vi "Qrcode Enum Page.vi"() -> ()   [LabVIEW 2019]
uses:
  <vilib>/userDefined/High Color/IMAQdx.ctl
  <vilib>/vision/driver/NI_Vision_Acquisition_Software.lvlib
  <vilib>/vision/NI_Vision_Development_Module.lvlib
panel:
  out "Page 2":string[](array[string])
  out "Page 1":string[](array[string])
  out "SIze Page 2":i32
  out "Size Page 1":i32
  out "Output Enum Data":enum16{"Page 1", "Page 2"}(ring)
  out "Index":i32
  in  "Enum Data":enum16{"Page 1", "Page 2"}[](array[ring])
  out "Data":string
  out "Array":string[](array[string])
  in  "Tab Control":enum32{"Data Qrcode", "Page 1", "Page 2"}(tab)
  out "Data Qrcode":string[](array[string])
  out "Found?":bool
  in  "Session In":T1
  out "Image":T2(plugin-control)
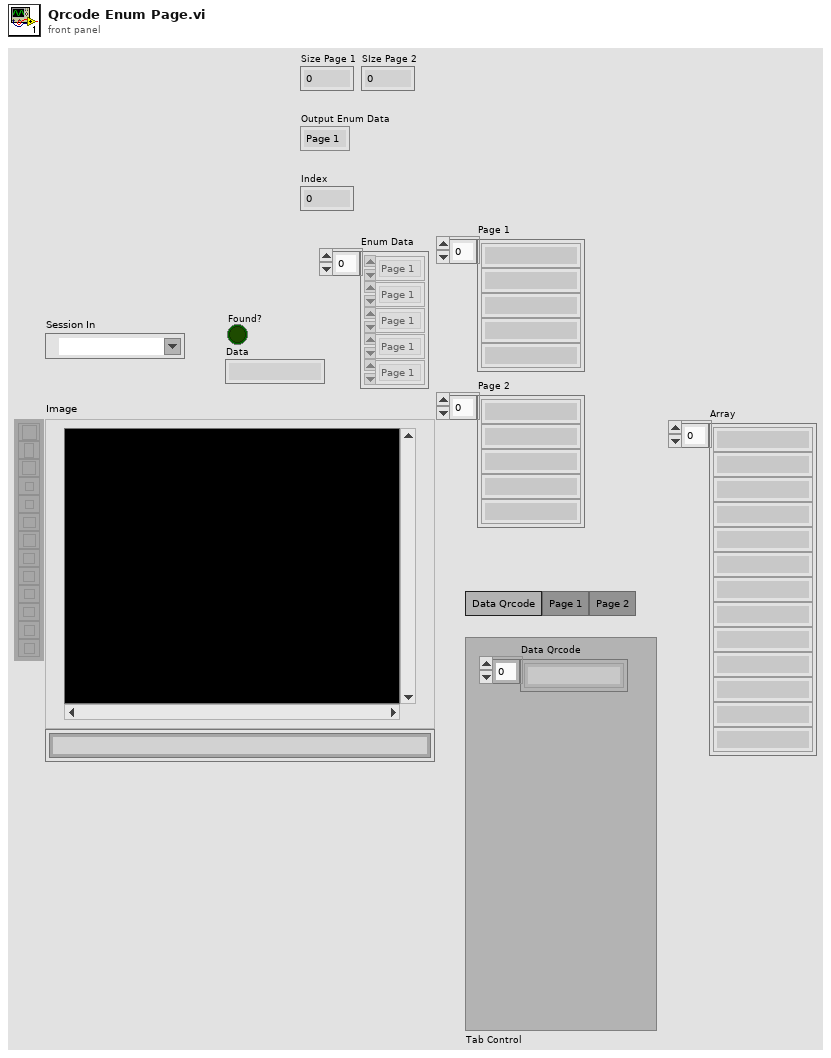
[diagram p1: front panel]
types:
  T1 = typedef "IMAQdx.ctl" = refnum<k21>
  T2 = typedef "IMAQ Image.ctl" = refnum<image>
  T3 = typedef "Image Type" = u32
  T4 = typedef "QR Code Report.ctl" = cluster{"Found?":bool, "Data":string, "Bounding Box":cluster{"x":sgl, "y":sgl}[], "Errors Corrected":u32, "Dimensions (Rows/Cols)":u32, "Version":u32, "QR Model":T5, "Stream Mode":T6, "Barcode Polarity":T7, "Mirrored?":bool, "Append Stream Position":u32, "Size of Append Stream":u32, "First EAN-128 ID":i32, "First Alternate Language ID":i32, "Append Stream ID":u32, "Minimum Edge Strength":u32, "Demodulation Mode":T8, "Cell Sample Size":T9, "Cell Filter Mode":T10}
  T5 = typedef "QR Code Model Type.ctl" = i32
  T6 = typedef "QR Code Stream Mode Type.ctl" = i32
  T7 = typedef "Data Matrix Polarity.ctl" = i32
  T8 = typedef "Demodulation Mode.ctl" = i32
  T9 = typedef "Cell Sample Size.ctl" = i32
  T10 = typedef "Cell Filter Mode.ctl" = i32
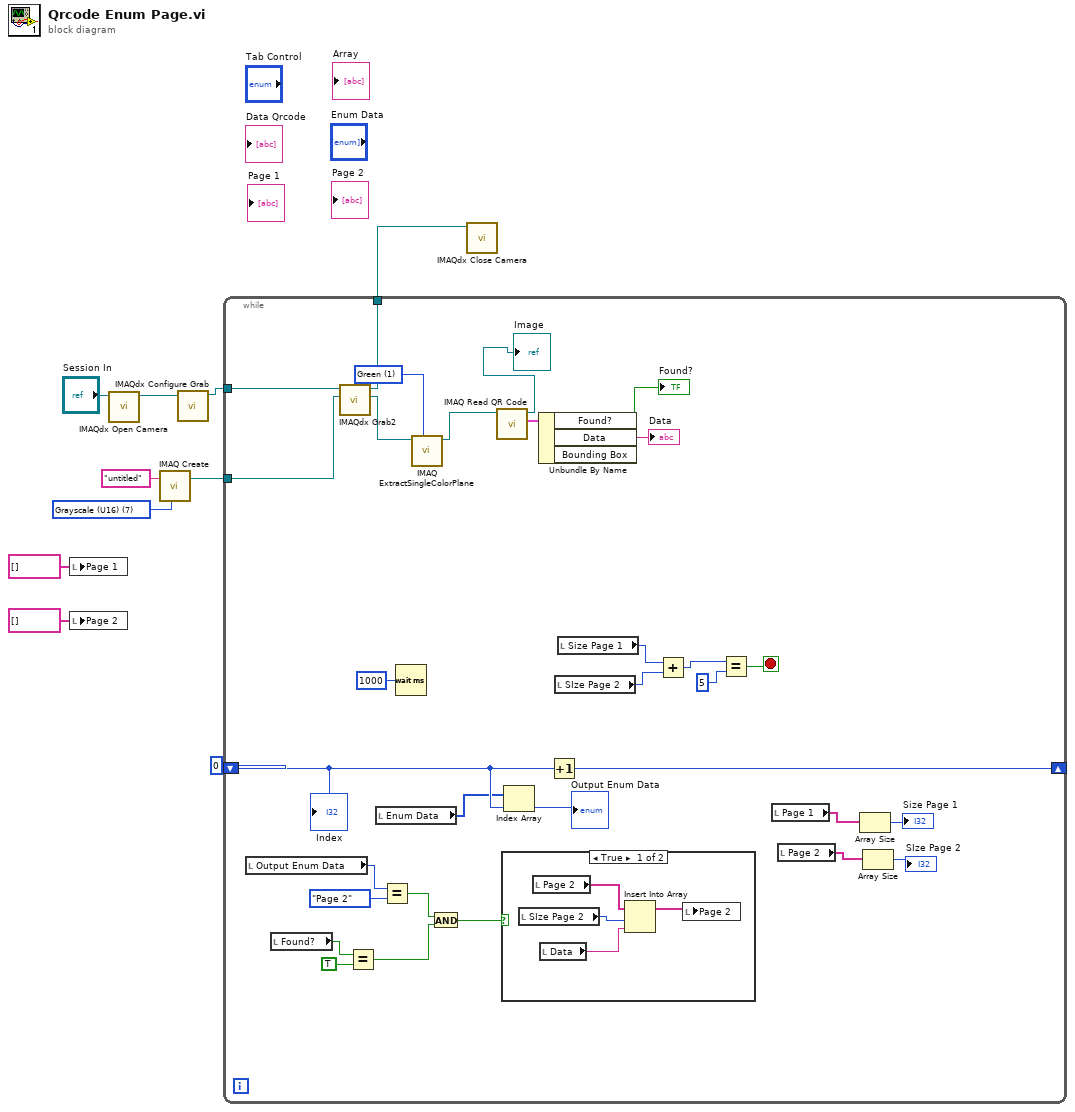
[diagram p0: block diagram]
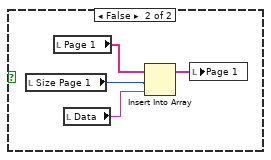
[diagram p2: hidden frame]
diagram:
  w9 = T3 7 items=["Grayscale (U8)", "Grayscale (I16)", "Grayscale (SGL)", "Complex (CSG)", "RGB (U32)", "HSL (U32)", "RGB (U64)", "Grayscale (U16)"] ("Image Type")
  n1 = local write "Page 1"(string[] [] ("Page 1")) -> ()
  n2 = local write "Page 2"(string[] [] ("Page 2")) -> ()
  n3 = call <vilib>:"IMAQdx Open Camera.vi"("Session In"="Session In") -> ("Session Out"=w8:T1)  [unwired: 9 in, 1 out]
  n4 = call "IMAQ Create"("Image Name"="untitled", "Image Type"=w9) -> ("New Image"=w5:T2)  [unwired: 3 in, 1 out]
  n5 = call <vilib>:"IMAQdx Configure Grab.vi"("Session In"=w8) -> ("Session Out"=w6:T1)  [unwired: 9 in, 1 out]
  n6 = while {
    tunnel: w6 -> [w41]
    tunnel: w5 -> [w40]
    tunnel: [w39] -> w4
    shift-right: [w31] -> _
    shift-left: 0 -> [w30]
    stop <- w21 stop-if-true
    w37 = 1 items=["Red", "Green", "Blue", "Hue", "Saturation", "Luminance", "Value", "Intensity"] ("Color Plane")
    n7 = local read "Output Enum Data"() -> (w15:enum16{"Page 1", "Page 2"})
    n8 = local read "Found?"() -> (w17:bool)
    n9 = call <vilib>:"IMAQdx Grab2.vi"("Image In"=w40, "Session In"=w41) -> ("Image Out"=w38:T2, "Session Out"=w39:T1)  [unwired: 6 in, 2 out]
    n10 = Equal?(x=w17, y=TRUE) -> (x = y?=w12:bool)
    n11 = local read "Enum Data"() -> (w29:enum16{"Page 1", "Page 2"}[])
    n12 = Equal?(x=w15, y=enum16{"Page 1", "Page 2"}."Page 2") -> (x = y?=w13:bool)
    n13 = Wait (ms)(milliseconds to wait=u32 1000) -> ()  [unwired: 1 out]
    n14 = call "IMAQ ExtractSingleColorPlane"("Color Plane"=w37, "Image Src"=w38) -> ("Image Dst Out"=w36:T2)  [unwired: 8 in, 1 out]
    n15 = And(x=w13, y=w12) -> (x .and. y?=w11:bool)
    n16 = call "IMAQ Read QR Code"("Image"=w36) -> ("QR Code Report"=w34:T4, "Image (duplicate)"=→"Image":T2)  [unwired: 7 in, 2 out]
    n17 = case shown="True" w11 {
      frame True {
        n18 = local read "SIze Page 2"() -> (w45:i32)
        n19 = local read "Page 2"() -> (w43:string[])
        n20 = local read "Data"() -> (w44:string)
        n21 = Insert Into Array(array=w43, index=w45, new element=w44) -> (w42:string[])
        n22 = local write "Page 2"(w42) -> ()
      }
      frame False {
        n23 = local read "Size Page 1"() -> (w49:i32)
        n24 = local read "Page 1"() -> (w46:string[])
        n25 = local read "Data"() -> (w48:string)
        n26 = Insert Into Array(array=w46, index=w49, new element=w48) -> (w47:string[])
        n27 = local write "Page 1"(w47) -> ()
      }
    }
    n28 = Index Array(array=w29, index=w30) -> (element=→"Output Enum Data":enum16{"Page 1", "Page 2"})
    n29 = Unbundle By Name(w34) -> ("Found?"=→"Found?":bool, "Data"=→"Data":string)  [unwired: 1 out]
    n30 = Increment(x=w30) -> (x+1=w31:i32)
    n31 = local read "SIze Page 2"() -> (w22:i32)
    n32 = local read "Size Page 1"() -> (w23:i32)
    n33 = Add(x=w23, y=w22) -> (x+y=w20:i32)
    n34 = Equal?(x=w20, y=5) -> (x = y?=w21:bool)
    n35 = local read "Page 1"() -> (w27:string[])
    n36 = local read "Page 2"() -> (w25:string[])
    n37 = Array Size(array=w27) -> (size(s)=→"Size Page 1":i32)
    n38 = Array Size(array=w25) -> (size(s)=→"SIze Page 2":i32)
    "Index" <- w30
  }
  n39 = call <vilib>:"IMAQdx Close Camera.vi"("Session In"=w4) -> ()  [unwired: 10 in, 1 out]
